vi "triton_controller.vi"(10 "Numerical Argument":dbl, 11 "Command":T1(ring)=enum."Read Heater Voltage") -> (3 "Response":string)   [LabVIEW 2021]
panel:
  # "TRITON CONTROLLER"
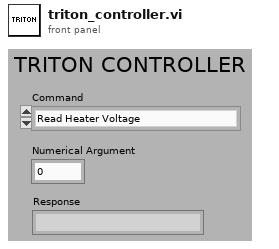
[diagram p1: front panel]
types:
  T1 = enum16{"Set Heater Voltage", "Read Heater Voltage", "Read Heater Current", "Read 1K Pot Temperature", "Read IVC Sorb Temperature", "Read Needle Valve Temperature", "Read Still Pressure", "Read Mixing Chamber Temperature", "Read STM RX Temperature", "Read STM CX Temperature", "Unstall Triton Loop", "Triton Stop", "Triton Stall Status"}
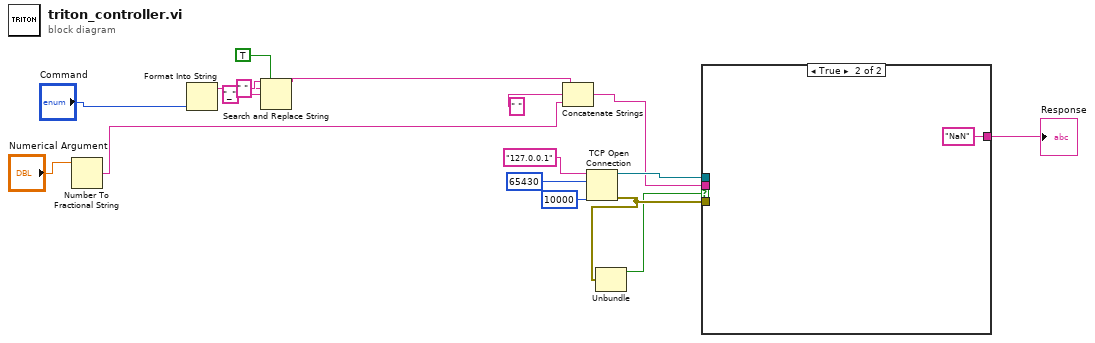
[diagram p0: block diagram]
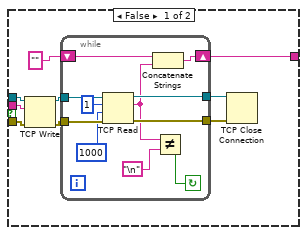
[diagram p2: hidden frame]
diagram:
  n1 = Number To Fractional String(number="Numerical Argument") -> (F-format string=w10:string)  [unwired: 3 in]
  n2 = Format Into String("Command") -> (resulting string=w9:string)  [unwired: 3 in, 1 out]
  n3 = Search and Replace String(replace all?=TRUE ("replace all? (F)"), input string=w9, search string=" ", replace string="_" ("replace string (\"\")")) -> (result string=w8:string)  [unwired: 4 in, 3 out]
  n4 = Concatenate Strings(w8, " " ("string"), w10) -> (w14:string)
  n5 = TCP Open Connection(address="127.0.0.1", remote port or service name=u16 65430, timeout ms (60000)=10000) -> (connection ID=w15:refnum<k5>, error out=w4:errorcluster)  [unwired: 2 in]
  n6 = Unbundle(w4) -> ("status"=w3:bool)  [unwired: 2 out]
  n7 = case shown="True" w3 {
    tunnel: w15 -> [w26 _]
    tunnel: w4 -> [w25 _]
    tunnel: w14 -> [w19 _]
    tunnel: [w18 "NaN" ("string")] -> w2
    frame False {
      n8 = TCP Write(connection ID=w26, data in=w19, error in (no error)=w25) -> (connection ID out=w23:refnum<k5>, error out=w24:errorcluster)  [unwired: 1 in, 1 out]
      n9 = while {
        tunnel: w24 -> [w37]
        tunnel: w23 -> [w36]
        tunnel: [w35] -> w22
        tunnel: [w34] -> w21
        shift-right: [w30] -> w18
        shift-left: "" ("string") -> [w31]
        stop <- w29 continue-if-true
        n10 = TCP Read(connection ID=w36, bytes to read=1, error in (no error)=w37, 9:1000 ("timeout ms (25000)")) -> (connection ID out=w34:refnum<k5>, data out=w28:string, error out=w35:errorcluster)  [unwired: 1 in]
        n11 = Concatenate Strings(w31, w28) -> (w30:string)
        n12 = Not Equal?(x=w28, y="\n") -> (x != y?=w29:bool)
      }
      n13 = TCP Close Connection(connection ID=w21, error in (no error)=w22) -> ()  [unwired: 1 in, 2 out]
    }
    frame True {
    }
  }
  "Response" <- w2
